vi "5GNR_DPD_AMPM_EVM_ACP_UL.vi"() -> ()   [LabVIEW 2016]
doc: "This example illustrates how to use the RFmx SpecAn and LTE personalities together with the RFSG drivers to perform ACP and EVM measurements with or without digital predistortion (DPD) of the waveform input to the DUT. \n\nDPD is a technique to optimize the operating point of power amplifiers and other non-linear RFIC devices. Power amplifiers are much more efficient if they operate near compression. However, compressing signal amplitudes can significantly deteriorate the amplified signal's quality both, in-band (e.g., EVM increases due to non-linear distortion of the signal's I/Q constellation) and out-of-band (e.g., ACP or SEM test fails due to spectral regrowth). With DPD, the original waveform is first pre-distorted in a way that matches the non-linear effects of the RFIC device before being fed through the device. The resulting output is a much cleaner amplified and/or filtered version of the original waveform. \n\nDifferent DPD models can be used to trade off performance with computational ease, with the Lookup-Table (LUT) model the simplest and the Generalized Memory Polynomial Model (GMP) the most complex. With a LUT, the DPD algorithm achieves gain and phase linearization on average. If you want to correct for memory effects - i.e., an output sample not only depends on the current input but also previous input samples; you will notice that a specific input power value translates into a range of gain and phase values - you would use one of the memory polynomial models. For these models, several parameters such as polynomial order and memory depth are available to fine-tune the model to the DUT behavior."
uses:
  <instrlib>/niRFSG/niRFSG.llb/niRFSG Exported Signal Destinations.ctl
  Source/SG/Typedefs/Instrument Configuration.ctl
  <instrlib>/niRFSG/niRFSG.llb/niRFSG Ref Clock Sources.ctl
  Source/Common/Local Oscillator Sharing Mode.ctl
  Source/Common/SA Common Configuration.ctl
  Source/SA/RFmxNR/Typedefs/NR ACP Configuration.ctl
  Source/SA/RFmxNR/Typedefs/NR ModAcc Configuration.ctl
  Source/SA/RFmxNR/Typedefs/NR ModAcc Component Carrier Results.ctl
  Source/SA/RFmxNR/Typedefs/NR ACP Offset Results.ctl
  Source/SA/RFmxNR/Typedefs/NR ACP Component Carrier Results.ctl
  Source/SA/RFmxSpecAn/Typedefs/SpecAn AMPM Results.ctl
  Source/SA/RFmxSpecAn/Typedefs/SpecAn AMPM Configuration.ctl
  Source/Common/Waveform.ctl
  Source/Methods/RFmxDPD/Typedefs/Memory Polynomial Configuration.ctl
  Source/Methods/RFmxDPD/Typedefs/Common Configuration.ctl
  Source/SA/RFmxInstr/Typedefs/Instrument Configuration.ctl
  Source/Methods/RFmxDPD/Typedefs/Pre DPD Crest Factor Reduction Configuration.ctl
  Source/Methods/RFmxDPD/Typedefs/Pre DPD Crest Factor Reduction Carrier Channel.ctl
  Source/Methods/RFmxDPD/Typedefs/Apply DPD Crest Factor Reduction Configuration.ctl
  Source/Common/SA Auto Level Configuration.ctl
  Source/SA/RFmxNR/Typedefs/NR Standard Configuration.ctl
  <vilib>/RFmx/SpecAn/mx/RFmxSpecAn.llb/RFmxSpecAn AMPM Fetch AM to AM Trace.vi
  <vilib>/RFmx/SpecAn/mx/RFmxSpecAn.llb/RFmxSpecAn AMPM Fetch AM to PM Trace.vi
  <vilib>/RFmx/NR/mx/RFmxNR.llb/RFmxNR ModAcc Fetch PUSCH Data Constellation Trace.vi
  <vilib>/RFmx/NR/mx/RFmxNR.llb/RFmxNR ModAcc Fetch PUSCH DMRS Constellation Trace.vi
  <vilib>/RFmx/NR/mx/RFmxNR.llb/RFmxNR ModAcc Fetch RMS EVM per Subcarrier Mean Trace.vi
  <vilib>/RFmx/NR/mx/RFmxNR.llb/RFmxNR ACP Fetch Relative Powers Trace.vi
  <vilib>/RFmx/NR/mx/RFmxNR.llb/RFmxNR ACP Fetch Spectrum.vi
  Source/SG/SG.lvlib
  Source/SA/RFmxNR/RFmxNR.lvlib
  Source/SA/RFmxSpecAn/RFmxSpecAn.lvlib
  Source/Methods/RFmxDPD/RFmxDPD.lvlib
  Source/SA/RFmxInstr/RFmxInstr.lvlib
  Source/Common/Common.lvlib
panel:
  in  "Center Frequency / SG IF (Hz)":dbl=3500000000.0 format="%.6p"
  in  "Error Tab Control":enum32{"Page 1", "Page 2"}(tab)
  out "error out":errorcluster
  in  "Display Tab Control":T1(tab)
  out "AM to AM Plot":T2(graph)
  out "AM to PM Plot":T3(graph)
  out "AMPM Measurement Results":T4 {"AM to PM Residual (deg)" format="%.2f"; "AM to AM Residual (dB)" format="%.2f"; "Mean RMS EVM (%)" format="%.2f"; "1 dB Compression Point (dBm)" format="%.2f"; "Mean Linear Gain (dB)" format="%.2f"}
  out "ModAcc Results":cluster{"Component Carrier Results":T5[]}
  out "Constellation Traces":cluster{"DMRS  Constellation":csg[]}[](graph)
  out "EVM Per Subcarrier Trace":cluster{"x0":dbl, "dx":dbl, "y":sgl[]}(graph)
  out "Spectrum":cluster{"x0":dbl, "dx":dbl, "y":sgl[]}[](graph)
  out "ACP Results":T8
  in  "Measurement Settings Tab Control":T9(tab)
  in  "RFmx SpecAn AMPM Configuration":T10={"Measurement Interval (s)"=0.0001, "DUT Average Input Power (dBm)"=-20.0, "Signal Type"=0, "Averaging Enabled"=0, "Averaging Count"=10, "Reference Waveform"={"Name"="Wfm", "Data"=refnum, "Signal Bandwidth (Hz)"=0.0, "PAPR (dB)"=0.0, "Burst Length (s)"=0.0, "Sample Rate"=0.0, "Burst Start Locations"=[], "Burst Stop Locations"=[], "Idle Duration Present?"=FALSE, "Runtime Scaling"=0.0, "Script"=""}} {"Reference Waveform"."Runtime Scaling" format="%#_6p"; "Reference Waveform"."Sample Rate" format="%#_6p"; "Reference Waveform"."Burst Length (s)" format="%#_6p"; "Reference Waveform"."PAPR (dB)" format="%.2f"; "Reference Waveform"."Signal Bandwidth (Hz)" format="%#_6p"; "Averaging Enabled" items=["False", "True"]; "Signal Type" items=["Modulated", "Tones"]; "DUT Average Input Power (dBm)" format="%.2f"; "Measurement Interval (s)" format="%.2p"}
  in  "Memory Polynomial Configuration":T12={"Correction Type"=0, "Number of Iterations"=1, " Order"=3, " Depth"=2, "Lead Order"=2, "Lag Order"=2, "Lead Memory Depth"=2, "Lag Memory Depth"=2, "Maximum Lead"=2, "Maximum Lag"=2} {"Number of Iterations" min=1; "Correction Type" items=["Magnitude and Phase", "Magnitude Only", "Phase Only"]}
  in  "Common DPD Configuration":T13={"Measurement Interval (s)"=0.0001, "Signal Type"=0, "DUT Average Input Power (dBm)"=-15.0, "Synchronization Method"=1} {"Synchronization Method" items=["Direct"=1, "Alias Protected"=2]; "DUT Average Input Power (dBm)" format="%.2f"; "Signal Type" items=["Modulated", "Tones"]; "Measurement Interval (s)" format="%#.2p"}
  in  "Enable DPD":bool=TRUE
  in  "Pre DPD Crest Factor Reduction":T14={"Enabled"=0, "Method"=0, "Max Iterations"=10, "Target PAPR (dB)"=8.0, "Shaping Factor"=5.0, "Shaping Threshold (dB)"=-5.0, "Window Type"=7, "Window Length"=10, "Filter Enabled"=0, "Carrier Channels"=[{"Offset (Hz)"=0.0, "Bandwidth (Hz)"=20000000.0}]} {"Carrier Channels"."Bandwidth (Hz)" format="%.2p"; "Carrier Channels"."Offset (Hz)" format="%.2p"; "Filter Enabled" items=["False", "True"]; "Window Type" items=["Flat Top"=1, "Hanning"=2, "Hamming"=3, "Gaussian"=4, "Blackman"=5, "Blackman-Harris"=6, "Kaiser-Bessel"=7]; "Method" items=["Clipping", "Peak Windowing", "Sigmoid"]; "Enabled" items=["False", "True"]}
  in  "Apply DPD Crest Factor Reduction":T16={"Enabled"=0, "Method"=0, "Max Iterations"=10, "Target PAPR Type"=0, "Target PAPR (dB)"=8.0, "Window Type"=7, "Window Length"=10, "Shaping Factor"=5.0, "Shaping Threshold (dB)"=-5.0} {"Target PAPR Type" items=["Input PAPR", "Custom"]; "Window Type" items=["Flat Top"=1, "Hanning"=2, "Hamming"=3, "Gaussian"=4, "Blackman"=5, "Blackman-Harris"=6, "Kaiser-Bessel"=7]; "Method" items=["Clipping", "Peak Windowing", "Sigmoid"]; "Enabled" items=["False", "True"]}
  in  "NR ModAcc Configuration":T17={"Measurement Length Unit"=1, "Measurement Offset"=0.0, "Measurement Length"=1.0, "EVM Unit"=0, "Averaging Enabled"=0, "Averaging Count"=10} {"Averaging Enabled" items=["False", "True"]; "EVM Unit" items=["Percentage", "dB"]; "Measurement Length Unit" items=["Slot"=1, "Subframe"=3, "Time"=6]}
  in  "NR ACP Configuration":T18={"Number of UTRA Offsets"=2, "Number of EUTRA Offsets"=0, "Number of NR Offsets"=2, "Number of ENDC Offsets"=0, "Measurement Method"=0, "Noise Compensation Enabled"=0, "Sweep Time Auto"=1, "Sweep Time Interval (s)"=0.001, "Averaging Enabled"=0, "Averaging Count"=10, "Averaging Type"=0} {"Measurement Method" items=["Normal", "Dynamic Range", "Sequential FFT"]; "Noise Compensation Enabled" items=["False", "True"]; "Sweep Time Auto" items=["False", "True"]; "Averaging Type" items=["RMS", "Log", "Scalar", "Max", "Min"]; "Averaging Enabled" items=["False", "True"]}
  in  "Resource Control":enum32{"RFSG", "5GNR Signal", "RFSA"}(tab)
  in  "Marker Event Output Terminal":T19="PXI_Trig0"
  in  "Reference Waveform File Path":path=path "C:/Users/Public/Documents/National Instruments/RFIC Test Software/Waveforms/NR_FR1_UL_1x100MHz_30kHz-SCS_256QAM_OS4_VST2_1ms.tdms"
  in  "RFSG Resource Name":refnum<k15>="5840"
  in  "SG Configuration":T20={"SelectedPorts"="", "Reference Clock Source"="PXI_CLK", "Carrier Frequency (Hz)"=3500000000.0, "DUT Average Input Power (dBm)"=-10.0, "External Attenuation (dB)"=0.0, "LO Sharing Mode"=enum."Automatic"}
  in  "Auto RB Detection Enabled":i32(ring)=1 items=["False", "True"]
  in  "Frequency Band":i32=78
  in  "Component Carrier Configurations":T23(array[cluster])=[{"Bandwidth (Hz)"=100000000.0, "Cell ID"=0, "PUSCH Modulation Type"=3, "Subcarrier Spacing (Hz)"=30000.0, "PUSCH Resource Block Offset"=0, "PUSCH Number of Resource Blocks"=-1}] {"Bandwidth (Hz)" items=["5M"=5000000.0, "10M"=10000000.0, "15M"=15000000.0, "20M"=20000000.0, "25M"=25000000.0, "30M"=30000000.0, "40M"=40000000.0, "50M"=50000000.0, "60M"=60000000.0, "70M"=70000000.0, "80M"=80000000.0, "90M"=90000000.0, "100M"=100000000.0, "200M"=200000000.0, "400M"=400000000.0]; "PUSCH Modulation Type" items=["PI/2 BPSK", "QPSK", "16 QAM", "64 QAM", "256 QAM"]; "Subcarrier Spacing (Hz)" items=["15kHz"=15000.0, "30kHz"=30000.0, "60kHz"=60000.0, "120kHz"=120000.0]}
  in  "SA RF (Hz)":dbl=nan format="%.6p"
  in  "RFSA Resource Name":refnum<k15>="5840"
  in  "Common Configuration":T24={"Center Frequency (Hz)"=3500000000.0, "Reference Level (dBm)"=0.0, "External Attenuation (dB)"=0.0, "Trigger Enabled"=TRUE, "Digital Trigger Source"="PXI_Trig0", "Trigger Delay (s)"=0.0, "Selected Ports"=""} {"Trigger Delay (s)" format="%.2p"; "External Attenuation (dB)" format="%.2f"; "Reference Level (dBm)" format="%.2f"; "Center Frequency (Hz)" format="%.6p"}
  in  "Instrument Configuration":T25={"LO Sharing Mode"=enum."Automatic", "Frequency Reference Source"="PXI_Clk"}
  in  "Auto Level Configuration":T26={"Enabled"=TRUE, "Measurement Interval (s)"=0.01} {"Measurement Interval (s)" min=1e-06 max=100.0 format="%.2p"}
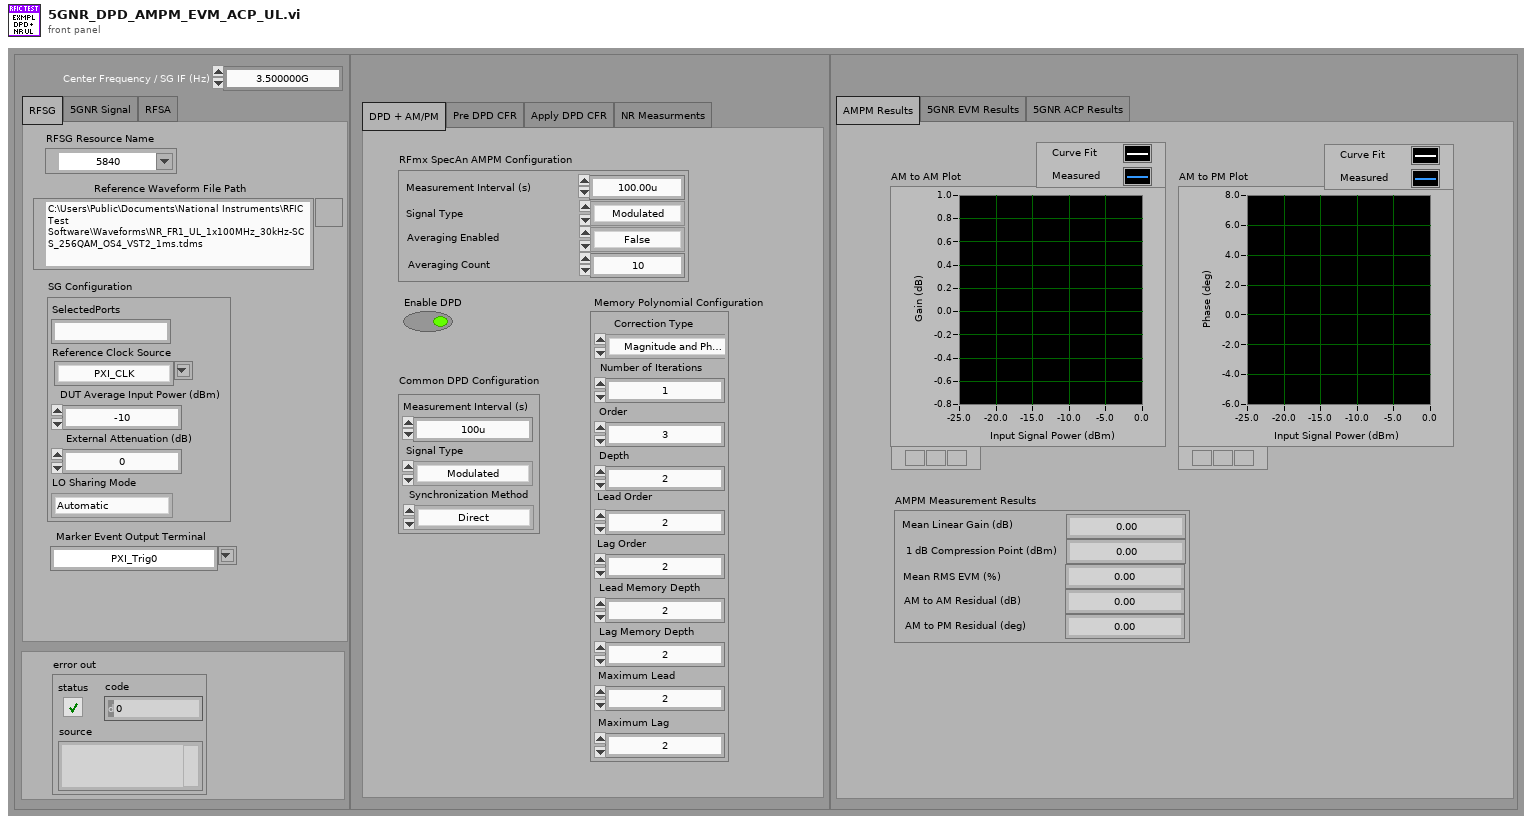
[diagram p1: front panel]
types:
  T1 = enum32{"AMPM Results", "5GNR EVM Results", "5GNR ACP Results"}
  T2 = cluster{"Input Powers (dBm)":sgl[], "Curve Fit AM to AM (dB)":sgl[]}[]
  T3 = cluster{"Input Powers (dBm)":sgl[], "Curve Fit AM to PM (dB)":sgl[]}[]
  T4 = typedef "RFmxSpecAn.lvlib/SpecAn AMPM Results.ctl" = cluster{"Mean Linear Gain (dB)":dbl, "1 dB Compression Point (dBm)":dbl, "Mean RMS EVM (%)":dbl, "AM to AM Residual (dB)":dbl, "AM to PM Residual (deg)":dbl}
  T5 = typedef "RFmxNR.lvlib/NR ModAcc Component Carrier Results.ctl" = cluster{"Peak Composite EVM Subcarrier Index":i32, "Peak Composite EVM Symbol Index":i32, "Mean RMS Composite EVM":dbl, "Max Peak Composite EVM":dbl, "Mean Frequency Error (Hz)":dbl, "Peak Composite EVM Slot Index":i32}
  T6 = typedef "RFmxNR.lvlib/NR ACP Offset Results.ctl" = cluster{"Upper Absolute Power (dBm)":dbl, "Lower Absolute Power (dBm)":dbl, "Lower Relative Power (dB)":dbl, "Upper Relative Power (dB)":dbl, "Frequency (Hz)":dbl, "Integration Bandwidth (Hz)":dbl}
  T7 = typedef "RFmxNR.lvlib/NR ACP Component Carrier Results.ctl" = cluster{"Absolute Power (dBm)":dbl, "Relative Power (dB)":dbl}
  T8 = cluster{"Offset Results":T6[], "Component Carrier Results":T7[]}
  T9 = enum32{"DPD + AM/PM", "Pre DPD CFR", "Apply DPD CFR", "NR Measurments"}
  T10 = typedef "RFmxSpecAn.lvlib/SpecAn AMPM Configuration.ctl" = cluster{"Measurement Interval (s)":dbl, "DUT Average Input Power (dBm)":dbl, "Signal Type":i32, "Averaging Enabled":i32, "Averaging Count":i32, "Reference Waveform":T11}
  T11 = typedef "Common.lvlib/Waveform.ctl" = cluster{"Name":string, "Data":refnum<data-value>, "Signal Bandwidth (Hz)":dbl, "PAPR (dB)":dbl, "Burst Length (s)":dbl, "Sample Rate":dbl, "Burst Start Locations":i32[], "Burst Stop Locations":i32[], "Idle Duration Present?":bool, "Runtime Scaling":dbl, "Script":string}
  T12 = typedef "RFmxDPD.lvlib/Memory Polynomial Configuration.ctl" = cluster{"Correction Type":i32, "Number of Iterations":i32, " Order":i32, " Depth":i32, "Lead Order":i32, "Lag Order":i32, "Lead Memory Depth":i32, "Lag Memory Depth":i32, "Maximum Lead":i32, "Maximum Lag":i32}
  T13 = typedef "RFmxDPD.lvlib/Common Configuration.ctl" = cluster{"Measurement Interval (s)":dbl, "Signal Type":i32, "DUT Average Input Power (dBm)":dbl, "Synchronization Method":i32}
  T14 = typedef "RFmxDPD.lvlib/Pre DPD Crest Factor Reduction Configuration.ctl" = cluster{"Enabled":i32, "Method":i32, "Max Iterations":i32, "Target PAPR (dB)":dbl, "Shaping Factor":dbl, "Shaping Threshold (dB)":dbl, "Window Type":i32, "Window Length":i32, "Filter Enabled":i32, "Carrier Channels":T15[]}
  T15 = typedef "RFmxDPD.lvlib/Pre DPD Crest Factor Reduction Carrier Channel.ctl" = cluster{"Offset (Hz)":dbl, "Bandwidth (Hz)":dbl}
  T16 = typedef "RFmxDPD.lvlib/Apply DPD Crest Factor Reduction Configuration.ctl" = cluster{"Enabled":i32, "Method":i32, "Max Iterations":i32, "Target PAPR Type":i32, "Target PAPR (dB)":dbl, "Window Type":i32, "Window Length":i32, "Shaping Factor":dbl, "Shaping Threshold (dB)":dbl}
  T17 = typedef "RFmxNR.lvlib/NR ModAcc Configuration.ctl" = cluster{"Measurement Length Unit":i32, "Measurement Offset":dbl, "Measurement Length":dbl, "EVM Unit":i32, "Averaging Enabled":i32, "Averaging Count":i32}
  T18 = typedef "RFmxNR.lvlib/NR ACP Configuration.ctl" = cluster{"Number of UTRA Offsets":i32, "Number of EUTRA Offsets":i32, "Number of NR Offsets":i32, "Number of ENDC Offsets":i32, "Measurement Method":i32, "Noise Compensation Enabled":i32, "Sweep Time Auto":i32, "Sweep Time Interval (s)":dbl, "Averaging Enabled":i32, "Averaging Count":i32, "Averaging Type":i32}
  T19 = typedef "niRFSG Exported Signal Destinations.ctl" = string
  T20 = typedef "SG.lvlib/Instrument Configuration.ctl" = cluster{"SelectedPorts":string, "Reference Clock Source":T21, "Carrier Frequency (Hz)":dbl, "DUT Average Input Power (dBm)":dbl, "External Attenuation (dB)":dbl, "LO Sharing Mode":T22}
  T21 = typedef "niRFSG Ref Clock Sources.ctl" = string
  T22 = typedef "Common.lvlib/Local Oscillator Sharing Mode.ctl" = enum16{"Automatic", "None"}
  T23 = cluster{"Bandwidth (Hz)":dbl, "Cell ID":i32, "PUSCH Modulation Type":i32, "Subcarrier Spacing (Hz)":dbl, "PUSCH Resource Block Offset":i32, "PUSCH Number of Resource Blocks":i32}[]
  T24 = typedef "Common.lvlib/SA Common Configuration.ctl" = cluster{"Center Frequency (Hz)":dbl, "Reference Level (dBm)":dbl, "External Attenuation (dB)":dbl, "Trigger Enabled":bool, "Digital Trigger Source":string, "Trigger Delay (s)":dbl, "Selected Ports":string}
  T25 = typedef "RFmxInstr.lvlib/Instrument Configuration.ctl" = cluster{"LO Sharing Mode":T22, "Frequency Reference Source":string}
  T26 = typedef "Common.lvlib/SA Auto Level Configuration.ctl" = cluster{"Enabled":bool, "Measurement Interval (s)":dbl}
  T27 = enum16{"ModAcc", "SEM", "ACP", "CHP", "OBW", "PVT"}[]
  T28 = enum16{"ACP", "CCDF", "CHP", "FCnt", "Harmonics", "OBW", "SEM", "Spectrum", "Spur", "TXP", "AMPM", "DPD", "IQ", "IM", "NF", "PhaseNoise", "PAVT"}[]
  T29 = typedef "RFmxNR.lvlib/NR Standard Configuration.ctl" = cluster{"Link Direction":i32, "Frequency Range":i32, "Band":i32, "Auto Resource Block Detection Enabled":i32, "Downlink Test Model":i32, "Downlink Test Model Duplex Scheme":i32, "Component Carrier Configurations":cluster{"Bandwidth (Hz)":dbl, "Cell ID":i32, "PUSCH Modulation Type":i32, "Subcarrier Spacing (Hz)":dbl, "PUSCH Resource Block Offset":i32, "PUSCH Number of Resource Blocks":i32, "PUSCH Transform Precoding Enabled":i32, "PUSCH Slot Allocation":string, "PUSCH Symbol Allocation":string, "PUSCH DMRS Configuration Type":i32, "PUSCH Mapping Type":i32, "PUSCH DMRS Type A Position":i32, "PUSCH DMRS Duration":i32, "PUSCH DMRS Additional Positions":i32}[]}
  T30 = cluster{"Bandwidth (Hz)":dbl, "Cell ID":i32, "PUSCH Modulation Type":i32, "Subcarrier Spacing (Hz)":dbl, "PUSCH Resource Block Offset":i32, "PUSCH Number of Resource Blocks":i32, "PUSCH Transform Precoding Enabled":i32, "PUSCH Slot Allocation":string, "PUSCH Symbol Allocation":string, "PUSCH DMRS Configuration Type":i32, "PUSCH Mapping Type":i32, "PUSCH DMRS Type A Position":i32, "PUSCH DMRS Duration":i32, "PUSCH DMRS Additional Positions":i32}
  T31 = cluster{"Reference Powers (dBm)":sgl[], "Curve Fit AM to AM (dB)":sgl[]}
  T32 = cluster{"Reference Powers (dBm)":sgl[], "Measured AM to AM (dB)":sgl[]}
  T33 = cluster{"Reference Powers (dBm)":sgl[], "Curve Fit AM to PM (deg)":sgl[]}
  T34 = cluster{"Reference Powers (dBm)":sgl[], "Measured AM to PM (deg)":sgl[]}
  T35 = cluster{"Reference Powers (dBm)":sgl[], "Measured AM to AM (dB)":sgl[]}[]
  T36 = cluster{"Reference Powers (dBm)":sgl[], "Measured AM to PM (deg)":sgl[]}[]
  T37 = typedef "RFmxNR.lvlib/NR ModAcc Results.ctl" = cluster{"Component Carrier Results":T5[]}
  T38 = typedef "RFmxNR.lvlib/NR ACP Results.ctl" = cluster{"Offset Results":T6[], "Component Carrier Results":T7[]}
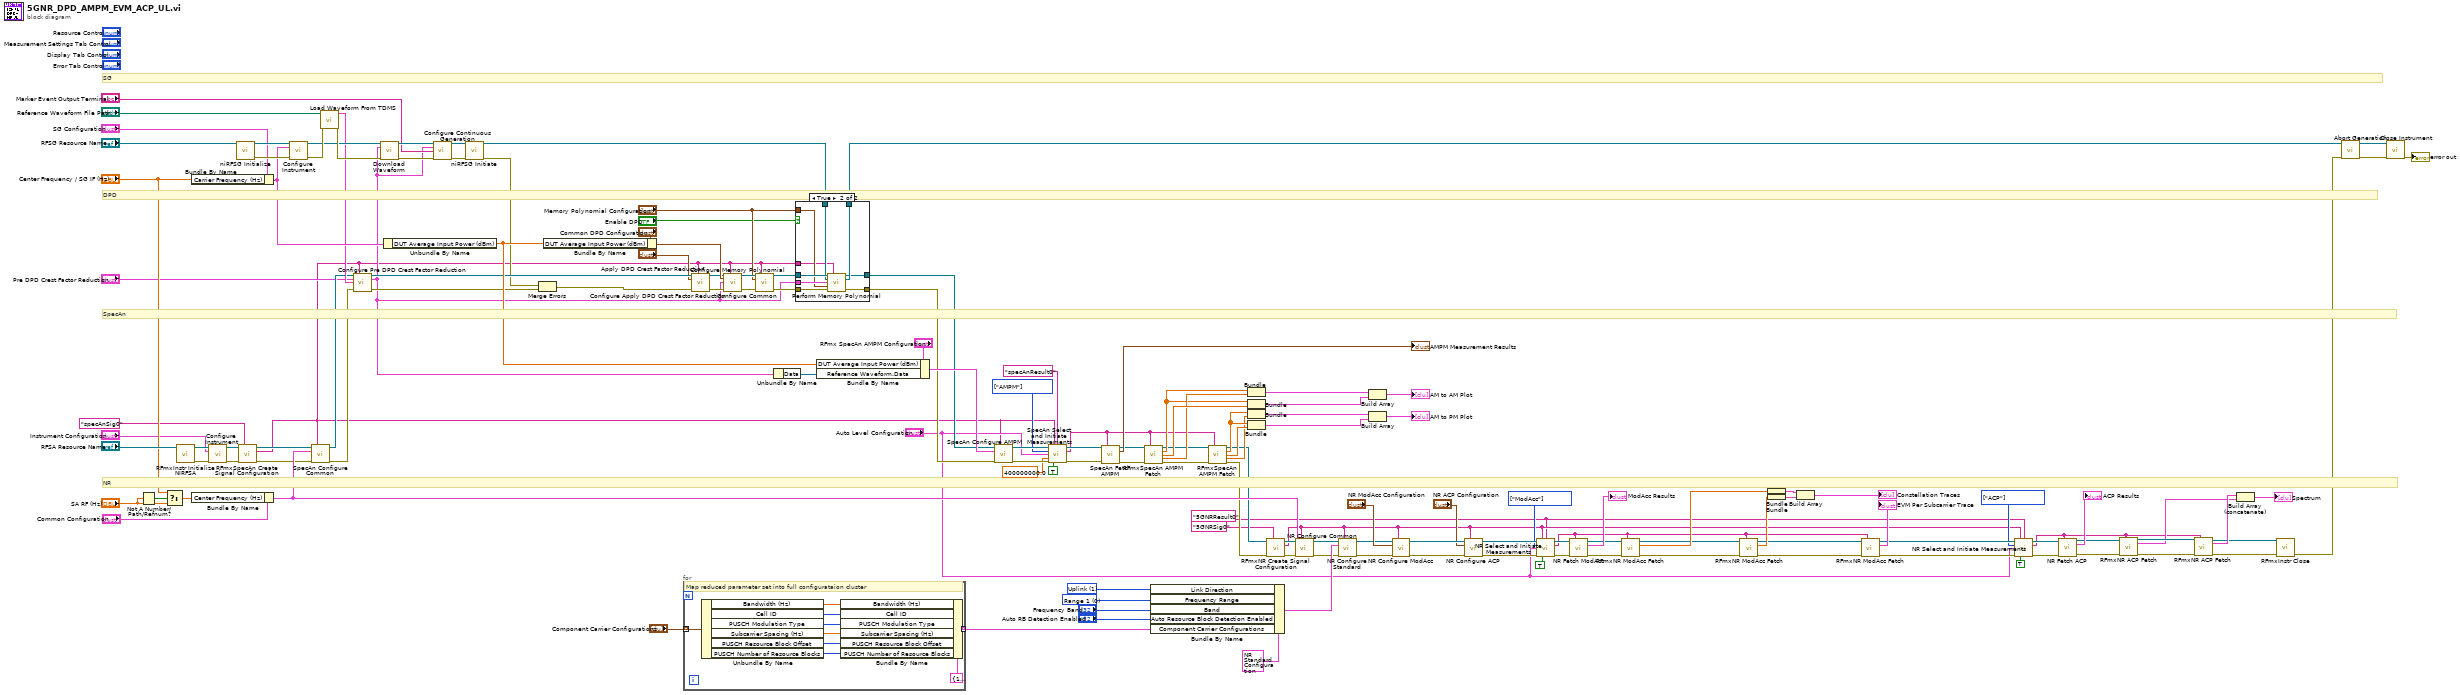
[diagram p0: block diagram]
diagram:
  w2 = "5GNRResult0"
  w23 = T27 [enum."ACP"] items=["ModAcc", "SEM", "ACP", "CHP", "OBW", "PVT"] ("Measurements")
  w30 = T27 [enum."ModAcc"] items=["ModAcc", "SEM", "ACP", "CHP", "OBW", "PVT"] ("Measurements")
  w36 = T28 [enum."AMPM"] items=["ACP", "CCDF", "CHP", "FCnt", "Harmonics", "OBW", "SEM", "Spectrum", "Spur", "TXP", "AMPM", "DPD", "IQ", "IM", "NF", "PhaseNoise", "PAVT"] ("Measurements")
  w137 = 0 items=["Range 1", "Range 2"] ("Frequency Range")
  w138 = 1 items=["Downlink", "Uplink"] ("Link Direction")
  # "SpecAn"
  # "SG"
  # "DPD"
  # "NR"
  n1 = Not A Number/Path/Refnum?(number/path/refnum="SA RF (Hz)") -> (NaN/Path/Refnum?=w141:bool)
  n2 = Select(t="Center Frequency / SG IF (Hz)", s=w141, f="SA RF (Hz)") -> (s? t:f=w123:dbl)
  n3 = call <vilib>:"RFmxInstr Initialize NIRFSA.vi"("Resource Name"="RFSA Resource Name") -> ("Instrument Handle Out"=w52:refnum<k21>, "error out"=w51:errorcluster)  [unwired: 12 in, 1 out]
  n4 = Bundle By Name(cluster="SG Configuration", "Carrier Frequency (Hz)"="Center Frequency / SG IF (Hz)") -> (w90:T20)
  n5 = Bundle By Name(cluster="Common Configuration", "Center Frequency (Hz)"=w123) -> (w53:T24)
  n6 = call "Configure Instrument.vi"("Instrument Handle In"=w52, "Instrument Configuration"="Instrument Configuration", "error in (no error)"=w51) -> ("Instrument Handle Out"=w20:refnum<k21>, "error out"=w17:errorcluster)  [unwired: 11 in]
  n7 = call <instrlib>:"niRFSG Initialize.vi"("resource name"="RFSG Resource Name") -> ("instrument handle"=w143:refnum<k15>, "error out"=w142:errorcluster)  [unwired: 13 in]
  n8 = call <vilib>:"RFmxSpecAn Create Signal Configuration.vi"("Instrument Handle In"=w20, "Signal Name"="specAnSig0", "error in (no error)"=w17) -> ("Instrument Handle Out"=w19:refnum<k21>, "Selector String Out"=w10:string, "error out"=w18:errorcluster)  [unwired: 10 in]
  n9 = call "Configure Instrument.vi"("RFSG Session In"=w143, "SG Configuration"=w90, "error in (no error)"=w142) -> ("RFSG Session Out"=w147:refnum<k15>, "error out"=w149:errorcluster)  [unwired: 11 in]
  n10 = call "SpecAn Configure Common.vi"("RFmx Handle In"=w19, "Selector String"=w10, "Common Configuration"=w53, "error in (no error)"=w18) -> ("RFmx Handle Out"=w44:refnum<k21>, "error out"=w43:errorcluster)  [unwired: 10 in]
  n11 = call "Load Waveform From TDMS.vi"("TDMS File Path"="Reference Waveform File Path", "error in (no error)"=w149) -> ("Waveform"=w45:T11, "error out"=w148:errorcluster)  [unwired: 12 in]
  n12 = call "Configure Pre DPD Crest Factor Reduction.vi"("Instrument Handle In"=w44, "Selector String"=w10, "Pre DPD Crest Factor Reduction Configuration"="Pre DPD Crest Factor Reduction", "Reference Waveform"=w45, "error in (no error)"=w43) -> ("Instrument Handle Out"=w47:refnum<k21>, "Pre DPD CFR Waveform"=w16:T11, "error out"=w46:errorcluster)  [unwired: 8 in]
  n13 = call "Download Waveform.vi"("RFSG handle"=w147, "Waveform In"=w16, "error in (no error)"=w148) -> ("RFSG handle out"=w132:refnum<k15>, "error out"=w130:errorcluster)  [unwired: 11 in]
  n14 = Unbundle By Name(w90) -> ("DUT Average Input Power (dBm)"=w57:dbl)
  n15 = call "Configure Continuous Generation.vi"("RFSG handle"=w132, "Waveform in"=w16, "Waveform Start Trigger Export"="Marker Event Output Terminal", "error in"=w130) -> ("RFSG handle out"=w131:refnum<k15>, "error out"=w129:errorcluster)  [unwired: 9 in, 1 out]
  n16 = call <instrlib>:"niRFSG Initiate.vi"("instrument handle"=w131, "error in"=w129) -> ("instrument handle out"=w64:refnum<k15>, "error out"=w14:errorcluster)  [unwired: 12 in]
  n17 = Merge Errors(w14, w46) -> (w15:errorcluster)
  n18 = Bundle By Name(cluster="Common DPD Configuration", "DUT Average Input Power (dBm)"=w57) -> (w58:T13)
  n19 = for {
    tunnel: [w157] -> w134 mode=indexing
    tunnel: "Component Carrier Configurations" -> [w156] mode=indexing
    # "Map reduced parameter set into full configurataion cluster"
    n20 = Unbundle By Name(w156) -> ("Bandwidth (Hz)"=w155:dbl, "Cell ID"=w154:i32, "PUSCH Modulation Type"=w153:i32, "Subcarrier Spacing (Hz)"=w152:dbl, "PUSCH Resource Block Offset"=w151:i32, "PUSCH Number of Resource Blocks"=w150:i32)
    n21 = Bundle By Name(cluster=T30 {"Bandwidth (Hz)"=100000000.0, "Cell ID"=0, "PUSCH Modulation Type"=1, "Subcarrier Spacing (Hz)"=30000.0, "PUSCH Resource Block Offset"=0, "PUSCH Number of Resource Blocks"=-1, "PUSCH Transform Precoding Enabled"=0, "PUSCH Slot Allocation"="0-Last", "PUSCH Symbol Allocation"="0-Last", "PUSCH DMRS Configuration Type"=0, "PUSCH Mapping Type"=0, "PUSCH DMRS Type A Position"=2, "PUSCH DMRS Duration"=1, "PUSCH DMRS Additional Positions"=0} ("NR Component Carrier Configuration"), "Bandwidth (Hz)"=w155, "Cell ID"=w154, "PUSCH Modulation Type"=w153, "Subcarrier Spacing (Hz)"=w152, "PUSCH Resource Block Offset"=w151, "PUSCH Number of Resource Blocks"=w150) -> (w157:T30)
  }
  n22 = call "Configure Apply DPD Crest Factor Reduction.vi"("Instrument Handle In"=w47, "Selector String"=w10, "Apply DPD Crest Factor Reduction Configuration"="Apply DPD Crest Factor Reduction", "error in (no error)"=w15) -> ("Instrument Handle Out"=w49:refnum<k21>, "error out"=w48:errorcluster)  [unwired: 10 in]
  n23 = call "Configure Common.vi"("Instrument Handle In"=w49, "Selector String"=w10, "Common Configuration"=w58, "Reference Waveform"=w16, "error in (no error)"=w48) -> ("Instrument Handle Out"=w66:refnum<k21>, "error out"=w65:errorcluster)  [unwired: 9 in]
  n24 = call "Configure Memory Polynomial.vi"("Instrument Handle In"=w66, "Selector String"=w10, "Memory Polynomial Configuration"="Memory Polynomial Configuration", "error in (no error)"=w65) -> ("Instrument Handle Out"=w67:refnum<k21>, "error out"=w68:errorcluster)  [unwired: 10 in]
  n25 = Unbundle By Name(w16) -> ("Data"=w56:refnum<data-value>)
  n26 = case shown="True" "Enable DPD" {
    tunnel: w67 -> [w160 w170]
    tunnel: [w159 w169] -> w54
    tunnel: "Memory Polynomial Configuration" -> [_ w163]
    tunnel: w16 -> [_ w168]
    tunnel: w64 -> [w161 w167]
    tunnel: [w161 w166] -> w63
    tunnel: [w160 w165] -> w55
    tunnel: w68 -> [w159 w164]
    tunnel: w10 -> [_ w162]
    frame False {
    }
    frame True {
      n27 = call "Perform Memory Polynomial.vi"("RFmx Instrument Handle In"=w170, "Selector String"=w162, "RFSG Instrument Handle In"=w167, "Reference Waveform"=w168, "Memory Polynomial Configuration"=w163, "error in (no error)"=w164) -> ("RFmx Instrument Handle Out"=w165:refnum<k21>, "RFSG Instrument Handle Out"=w166:refnum<k15>, "error out"=w169:errorcluster)  [unwired: 6 in, 1 out]
    }
  }
  n28 = Bundle By Name(cluster="RFmx SpecAn AMPM Configuration", "DUT Average Input Power (dBm)"=w57, "Reference Waveform.Data"=w56) -> (w87:T10)
  n29 = call "SpecAn Configure AMPM.vi"("RFmx Handle In"=w55, "Selector String"=w10, "RFmx SpecAn AMPM Configuration"=w87, "error in (no error)"=w54) -> ("RFmx Handle Out"=w40:refnum<k21>, "error out"=w39:errorcluster)  [unwired: 10 in]
  n30 = call "SpecAn Select and Initiate Measurements.vi"("Instrument Handle In"=w40, "Selector String"=w10, "Result Name"="specAnResult0", "Measurements"=w36, "Auto Level Configuration"="Auto Level Configuration", "Auto Level Bandwidth (Hz)"=400000000.0, "error in (no error)"=w39, "Enable All Traces (F)"=TRUE) -> ("Instrument Handle Out"=w38:refnum<k21>, "Selector String Out"=w12:string, "error out"=w37:errorcluster)  [unwired: 5 in]
  n31 = call "SpecAn Fetch AMPM.vi"("RFmx Handle In"=w38, "Selector String"=w12, "error in (no error)"=w37) -> ("RFmx Handle Out"=w71:refnum<k21>, "AMPM Results"=→"AMPM Measurement Results":T4, "error out"=w70:errorcluster)  [unwired: 10 in]
  n32 = call-poly <vilib>:"RFmxSpecAn AMPM Fetch.vi"("Instrument Handle In"=w71, "Selector String"=w12, "error in (no error)"=w70) -> ("Instrument Handle Out"=w79:refnum<k21>, "Reference Powers (dBm)"=w83:sgl[], "Measured AM to AM (dB)"=w85:sgl[], "Curve Fit AM to AM (dB)"=w84:sgl[], "error out"=w78:errorcluster)  [unwired: 8 in]
  n33 = Bundle By Name(cluster=T29 {"Link Direction"=1, "Frequency Range"=0, "Band"=78, "Auto Resource Block Detection Enabled"=1, "Downlink Test Model"=0, "Downlink Test Model Duplex Scheme"=0, "Component Carrier Configurations"=[{"Bandwidth (Hz)"=100000000.0, "Cell ID"=0, "PUSCH Modulation Type"=1, "Subcarrier Spacing (Hz)"=30000.0, "PUSCH Resource Block Offset"=0, "PUSCH Number of Resource Blocks"=-1, "PUSCH Transform Precoding Enabled"=0, "PUSCH Slot Allocation"="0-Last", "PUSCH Symbol Allocation"="0-Last", "PUSCH DMRS Configuration Type"=0, "PUSCH Mapping Type"=0, "PUSCH DMRS Type A Position"=2, "PUSCH DMRS Duration"=1, "PUSCH DMRS Additional Positions"=0}]} ("NR Signal Configuration"), "Link Direction"=w138, "Frequency Range"=w137, "Band"="Frequency Band", "Auto Resource Block Detection Enabled"="Auto RB Detection Enabled", "Component Carrier Configurations"=w134) -> (w139:T29)
  n34 = call-poly <vilib>:"RFmxSpecAn AMPM Fetch.vi"("Instrument Handle In"=w79, "Selector String"=w12, "error in (no error)"=w78) -> ("Instrument Handle Out"=w9:refnum<k21>, "Reference Powers (dBm)"=w82:sgl[], "Measured AM to PM (deg)"=w81:sgl[], "Curve Fit AM to PM (deg)"=w80:sgl[], "error out"=w8:errorcluster)  [unwired: 8 in]
  n35 = Bundle("Reference Powers (dBm)"=w83, "Curve Fit AM to AM (dB)"=w84) -> (w77:T31)  [unwired: 1 in]
  n36 = Bundle("Reference Powers (dBm)"=w83, "Measured AM to AM (dB)"=w85) -> (w76:T32)  [unwired: 1 in]
  n37 = Bundle("Reference Powers (dBm)"=w82, "Curve Fit AM to PM (deg)"=w80) -> (w74:T33)  [unwired: 1 in]
  n38 = Bundle("Reference Powers (dBm)"=w82, "Measured AM to PM (deg)"=w81) -> (w75:T34)  [unwired: 1 in]
  n39 = call <vilib>:"RFmxNR Create Signal Configuration.vi"("Instrument Handle In"=w9, "Signal Name"="5GNRSig0", "error in (no error)"=w8) -> ("Instrument Handle Out"=w7:refnum<k21>, "Selector String Out"=w3:string, "error out"=w6:errorcluster)  [unwired: 10 in]
  n40 = call "NR Configure Common.vi"("RFmx Handle In"=w7, "Selector String"=w3, "Common Configuration"=w53, "error in (no error)"=w6) -> ("RFmx Handle Out"=w62:refnum<k21>, "error out"=w69:errorcluster)  [unwired: 10 in]
  n41 = call "NR Configure Standard.vi"("RFmx Handle In"=w62, "Selector String"=w3, "NR Standard Configuration"=w139, "error in (no error)"=w69) -> ("RFmx Handle Out"=w88:refnum<k21>, "error out"=w89:errorcluster)  [unwired: 10 in]
  n42 = Build Array(w77, w76) -> (→"AM to AM Plot":T35)
  n43 = Build Array(w74, w75) -> (→"AM to PM Plot":T36)
  n44 = call "NR Configure ModAcc.vi"("RFmx Handle In"=w88, "Selector String"=w3, "NR ModAcc Configuration"="NR ModAcc Configuration", "error in (no error)"=w89) -> ("RFmx Handle Out"=w128:refnum<k21>, "error out"=w127:errorcluster)  [unwired: 10 in]
  n45 = call "NR Configure ACP.vi"("RFmx Handle In"=w128, "Selector String"=w3, "NR ACP Configuration"="NR ACP Configuration", "error in (no error)"=w127) -> ("RFmx Handle Out"=w34:refnum<k21>, "error out"=w33:errorcluster)  [unwired: 10 in]
  n46 = call "NR Select and Initiate Measurements.vi"("Instrument Handle In"=w34, "Selector String"=w3, "Result Name"=w2, "Measurements"=w30, "Auto Level Configuration"="Auto Level Configuration", "error in (no error)"=w33, "Enable All Traces (F)"=TRUE) -> ("Instrument Handle Out"=w32:refnum<k21>, "Selector String Out"=w4:string, "error out"=w31:errorcluster)  [unwired: 6 in]
  n47 = call "NR Fetch ModAcc.vi"("RFmx Handle In"=w32, "Selector String"=w4, "error in (no error)"=w31) -> ("RFmx Handle Out"=w94:refnum<k21>, "ModAcc Results"=→"ModAcc Results":T37, "error out"=w93:errorcluster)  [unwired: 10 in]
  n48 = call-poly <vilib>:"RFmxNR ModAcc Fetch.vi"("Instrument Handle In"=w94, "Selector String"=w4, "error in (no error)"=w93) -> ("Instrument Handle Out"=w111:refnum<k21>, "PUSCH Data Constellation"=w114:csg[], "error out"=w112:errorcluster)  [unwired: 10 in]
  n49 = call-poly <vilib>:"RFmxNR ModAcc Fetch.vi"("Instrument Handle In"=w111, "Selector String"=w4, "error in (no error)"=w112) -> ("Instrument Handle Out"=w109:refnum<k21>, "PUSCH DMRS Constellation"=w113:csg[], "error out"=w110:errorcluster)  [unwired: 10 in]
  n50 = Bundle("PUSCH Data Constellation"=w114) -> (w116:cluster{"PUSCH Data Constellation":csg[]})  [unwired: 1 in]
  n51 = Bundle("PUSCH DMRS Constellation"=w113) -> (w107:cluster{"PUSCH DMRS Constellation":csg[]})  [unwired: 1 in]
  n52 = Build Array(w116, w107) -> (→"Constellation Traces":cluster{"PUSCH DMRS Constellation":csg[]}[])
  n53 = call-poly <vilib>:"RFmxNR ModAcc Fetch.vi"("Instrument Handle In"=w109, "Selector String"=w4, "error in (no error)"=w110) -> ("Instrument Handle Out"=w27:refnum<k21>, "RMS EVM per Subcarrier Mean (% or dB)"=→"EVM Per Subcarrier Trace":cluster{"x0":dbl, "dx":dbl, "y":sgl[]}, "error out"=w25:errorcluster)  [unwired: 10 in]
  n54 = call "NR Select and Initiate Measurements.vi"("Instrument Handle In"=w27, "Selector String"=w3, "Result Name"=w2, "Measurements"=w23, "Auto Level Configuration"="Auto Level Configuration", "error in (no error)"=w25, "Enable All Traces (F)"=TRUE) -> ("Instrument Handle Out"=w26:refnum<k21>, "Selector String Out"=w1:string, "error out"=w24:errorcluster)  [unwired: 6 in]
  n55 = call "NR Fetch ACP.vi"("RFmx Handle In"=w26, "Selector String"=w1, "error in (no error)"=w24) -> ("RFmx Handle Out"=w99:refnum<k21>, "ACP Results"=→"ACP Results":T38, "error out"=w98:errorcluster)  [unwired: 10 in]
  n56 = call-poly <vilib>:"RFmxNR ACP Fetch.vi"("Instrument Handle In"=w99, "Selector String"=w1, "error in (no error)"=w98) -> ("Instrument Handle Out"=w104:refnum<k21>, "Relative Powers (dB)"=w101:cluster{"x0":dbl, "dx":dbl, "y":sgl[]}[], "error out"=w103:errorcluster)  [unwired: 10 in]
  n57 = call-poly <vilib>:"RFmxNR ACP Fetch.vi"("Instrument Handle In"=w104, "Selector String"=w1, "error in (no error)"=w103) -> ("Instrument Handle Out"=w97:refnum<k21>, "Spectrum (dBm)"=w102:cluster{"x0":dbl, "dx":dbl, "y":sgl[]}, "error out"=w96:errorcluster)  [unwired: 10 in]
  n58 = Build Array (concatenate)(w102, w101) -> (→"Spectrum":cluster{"x0":dbl, "dx":dbl, "y":sgl[]}[])
  n59 = call <vilib>:"RFmxInstr Close.vi"("Instrument Handle In"=w97, "error in (no error)"=w96) -> ("error out"=w95:errorcluster)  [unwired: 13 in]
  n60 = call "Abort Generation.vi"("RFSG handle"=w63, "error in (no error)"=w95) -> ("RFSG handle out"=w146:refnum<k15>, "error out"=w145:errorcluster)  [unwired: 12 in]
  n61 = call "Close Instrument.vi"("RFSG Handle"=w146, "error in (no error)"=w145) -> ("error out"=→"error out":errorcluster)  [unwired: 13 in]
